vi "Hitrap_DiagnosticBoxGUI.panel.vi"() -> ()   [LabVIEW 2014, in "Hitrap_DiagnosticBoxGUI.lvlib"]
doc: "GUI for the DiagnosticBox class. It can be selected different step motors and perform a reference move to different diagnostics."
uses:
  Hitrap_DiagnosticBoxGUI.lvlib
  CSlibraries-extern/DimLVEvent/LVDimInterface/LVDimInterface.dim service type.ctl
  CSlibraries-extern/DimLVEvent/LVDimInterface/LVDimInterface.dic_info_service_notifier.vi
  CSCore/CSSystem/CoreLib/CoreLib.byte array 2 string.vi
  CSCore/CSSystem/CoreLib/CoreLib.int 2 byte array.vi
  CSCore/CSSystem/CoreLib/CoreLib.double 2 byte array.vi
  CSCore/CSSystem/CoreLib/CoreLib.lvlib
  CSlibraries/UtilityLib/UtilityLib.lvlib
  CSCore/GUIs/GOGUserGUIs/DeviceBaseGUI/DeviceBaseGUI.lvlib
  CSlibraries-extern/DimLVEvent/LVDimInterface/LVDimInterface.lvlib
  CSCore/BaseProcess/BaseProcess.lvlib
  CSCore/CSSystem/CSSystemLib/CSSystemLib.lvlib
panel:
  out "EMStop":bool
  out "loop 2":i32
  out "error out":errorcluster
  out "device state":bool
  out "error":bool=TRUE
  out "status":string
  out "pos error":bool
  out "status bit":u32(ring) items=["motorEnabled"=1, "negativeLimitSwitchActive"=2, "positiveLimitSwitchActive"=4, "limitSwitchesEnabled"=8, "limitSwitchesAreNormallyClosed"=16, "moving"=32, "referenced"=64, "inPosition"=128, "reserved2"=256, "reserved3"=512, "reserved4"=1024, "reserved5"=2048, "error"=4096, "reserved6"=8192, "reserved7"=16384, "reserved8"=32768, "user defined1"=65536, "user defined2"=131072, "user defined3"=262144, "user defined4"=524288, "user defined5"=1048576, "user defined6"=2097152, "user defined7"=4194304, "user defined8"=8388608, "user defined9"=16777216, "user defined10"=33554432, "user defined11"=67108864, "user defined12"=134217728, "user defined13"=268435456, "user defined14"=536870912, "user defined15"=1073741824, "user defined16"=2147483648]
  in  "Go Absolute":bool
  out "Moving":bool
  out "in Position":bool
  in  "steps to go":dbl
  out "loop 1":i32
  in  "error in (no error)":errorcluster
  in  "object ref":refnum<vi>
  in  "reset pos error":bool
  in  "Stop Movement":bool
  out "step count":dbl
  in  "Go Relative":bool
  out "Pos4Reached":bool
  in  "GoPosition4":bool
  in  "clear error":bool
  out "Enable":bool
  out "Pos3Reached":bool
  out "Pos2Reached":bool
  out "Pos1Reached":bool
  in  "GoPosition3":bool
  in  "GoPosition2":bool
  in  "GoPosition1":bool
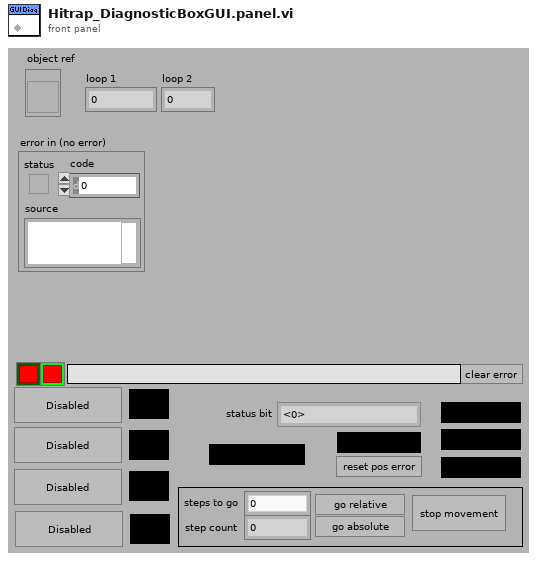
[diagram p1: front panel]
types:
  T1 = typedef "DeviceBaseGUI.lvlib/DeviceBaseGUI.i attribute.ctl" = cluster{"GOGFrontPanel.i attribute":T2}
  T2 = typedef "GOGFrontPanel.lvlib/GOGFrontPanel.i attribute.ctl" = cluster{"GOGObject":string, "Object":string, "Method":string, "Descriptor":T3, "Input Descriptor":string, "Output Descriptor":string, "inputNames":string[], "outputNames":string[], "Values":cluster{"descriptor":string, "value":string}[]}
  T3 = typedef "BaseProcess.lvlib/BaseProcess.descriptor string definition.ctl" = string
  T4 = cluster{"Diagnostic 1":string, "Diagnostic 2":string, "Diagnostic 3":string, "Diagnostic 4":string, "Diagnostic 5":string, "Position 1":dbl, "Position 2":dbl, "Position 3":dbl, "Position 4":dbl, "Position 5":dbl, "Reverse?":bool}
  T5 = enum8{"Enabled", "Disabled", "Disabled and Grayed Out"}
  T6 = typedef "LVDimInterface.lvlib/LVDimInterface.dim service type.ctl" = u16
  T7 = typedef "CoreDefs.call_type.ctl" = cluster{"Object":string, "Selector":string, "CallType":enum16{"simple", "synchronous", "asynchronous"}, "Async Object":string, "Async Selector":string, "Data Descriptor":T3, "Data":T8, "Error #":i32, "Expire":u32}
  T8 = typedef "CoreDefs.rawDataType.ctl" = i8[]
  T9 = typedef "MotorBase.lvlib/MotorBase.statusType.ctl" = u32
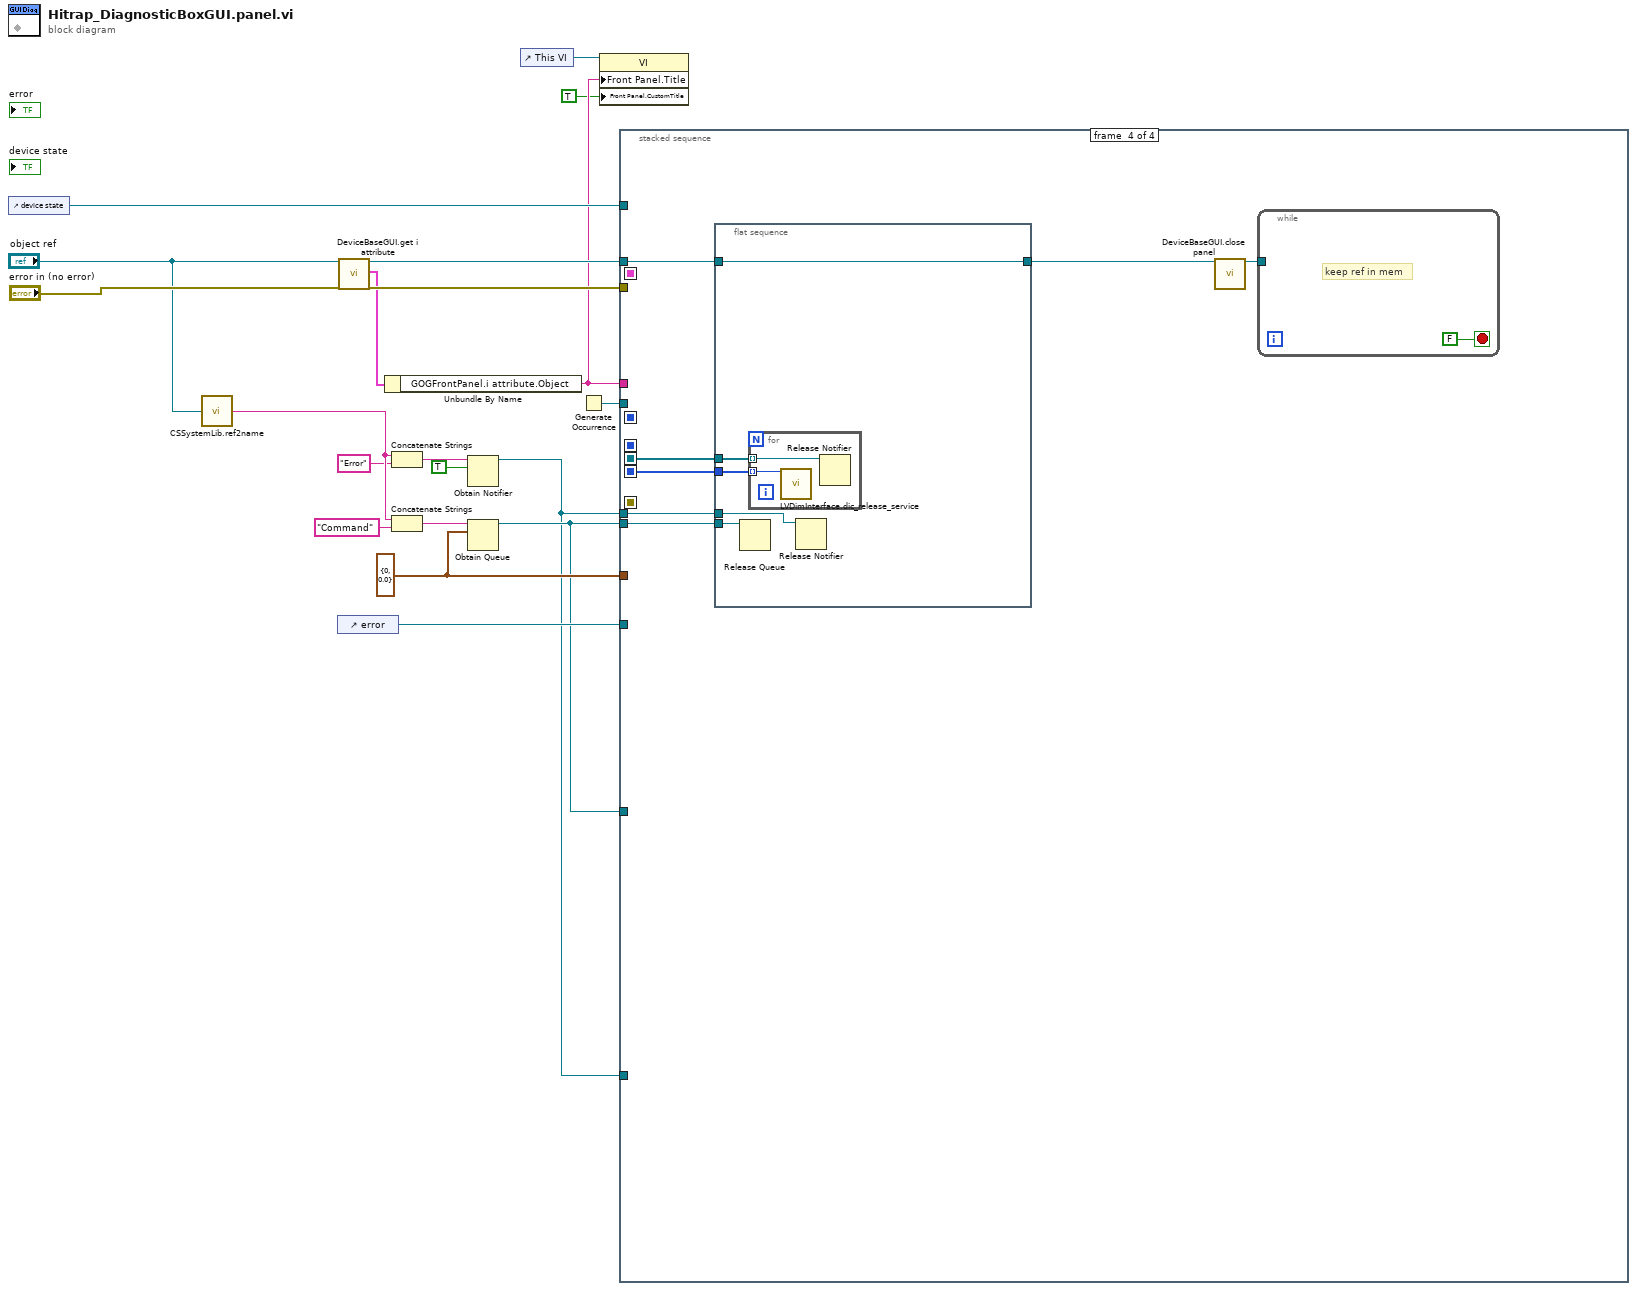
[diagram p0: block diagram]
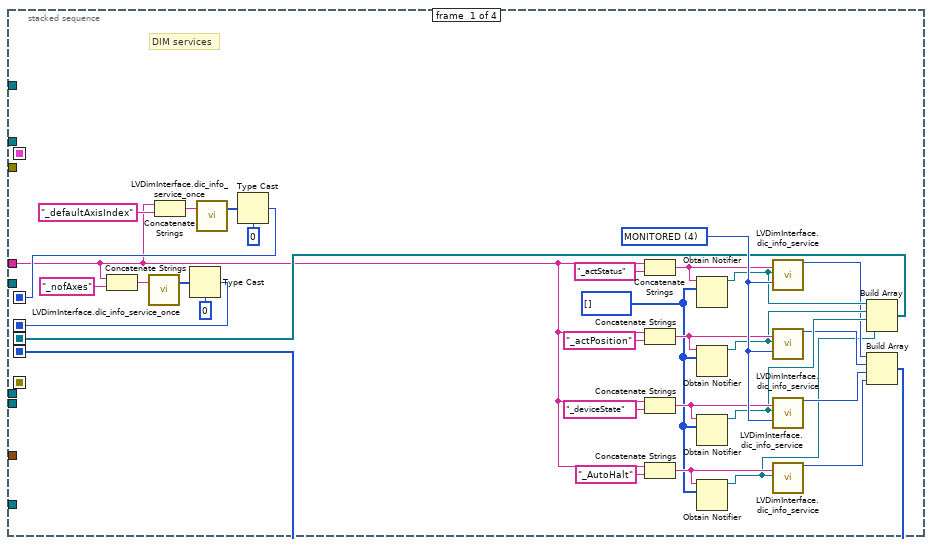
[diagram p2: hidden frame]
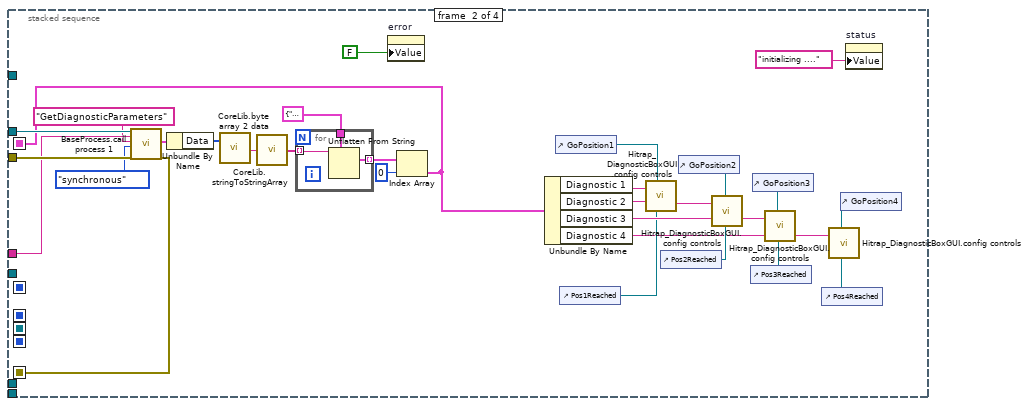
[diagram p3: hidden frame]
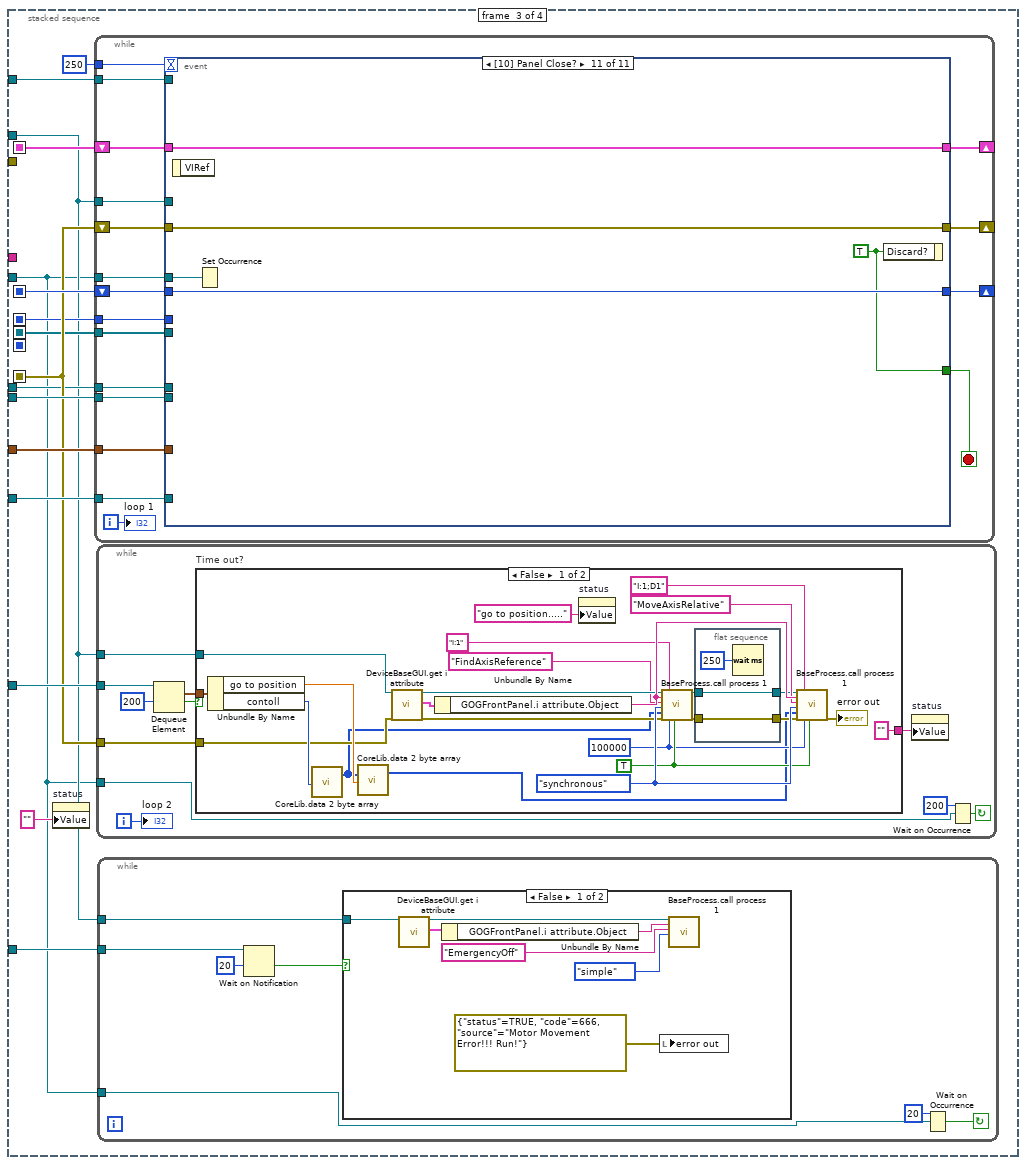
[diagram p4: hidden frame]
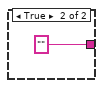
[diagram p6: hidden frame]
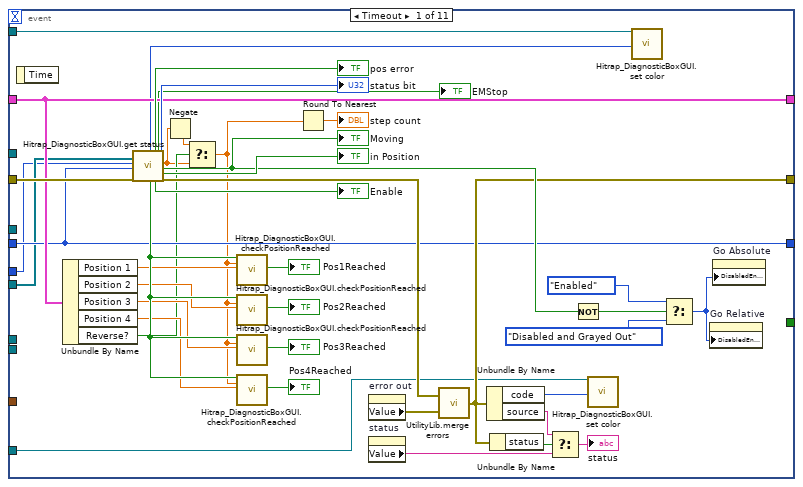
[diagram p7: hidden frame]
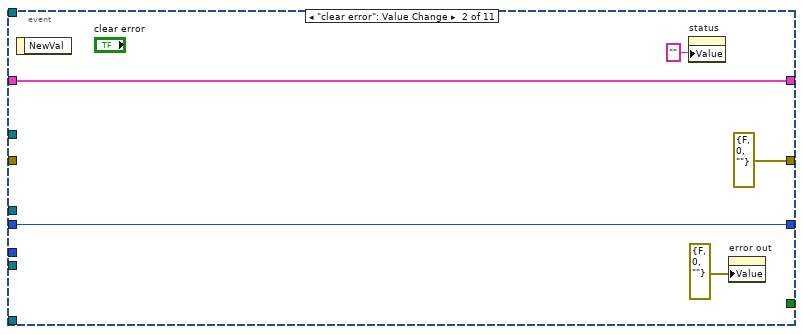
[diagram p8: hidden frame]
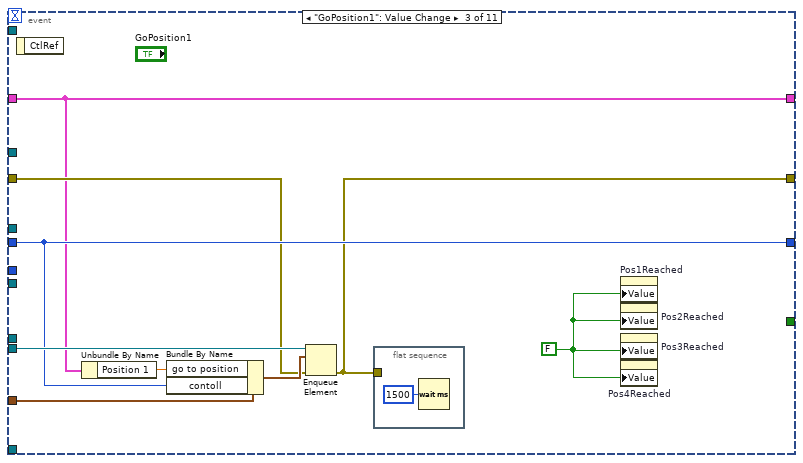
[diagram p9: hidden frame]
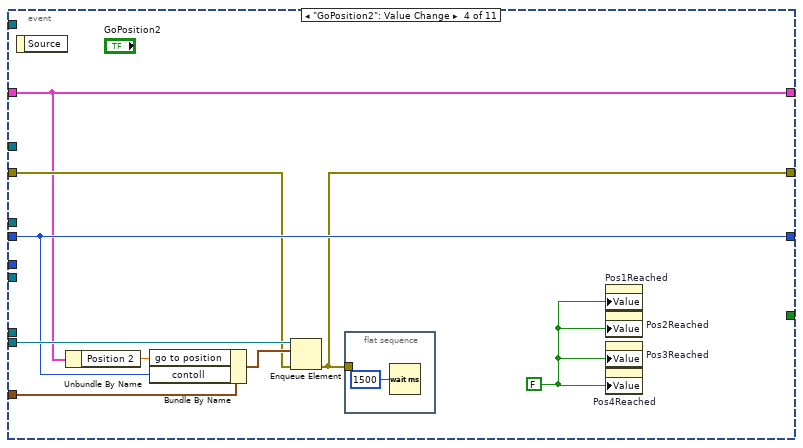
[diagram p10: hidden frame]
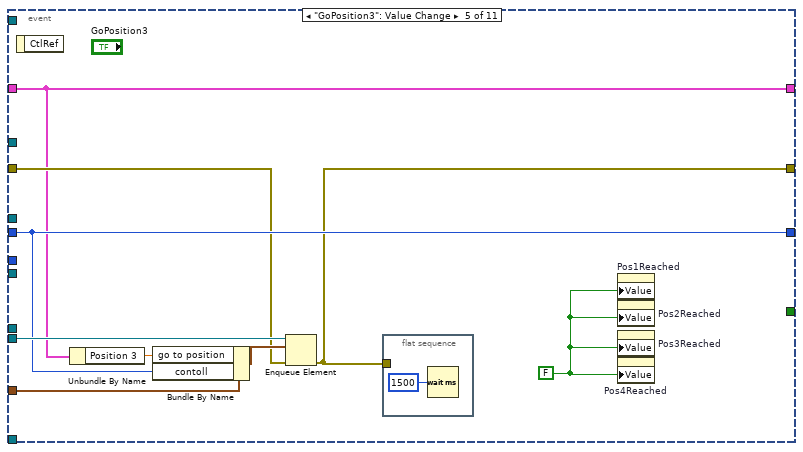
[diagram p11: hidden frame]
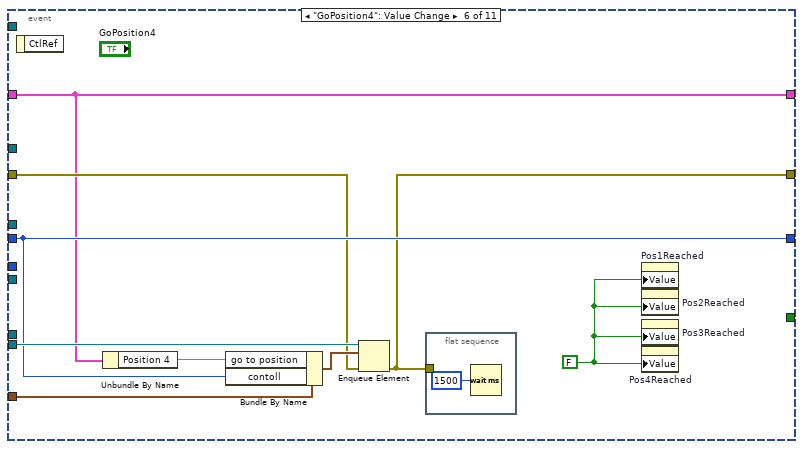
[diagram p12: hidden frame]
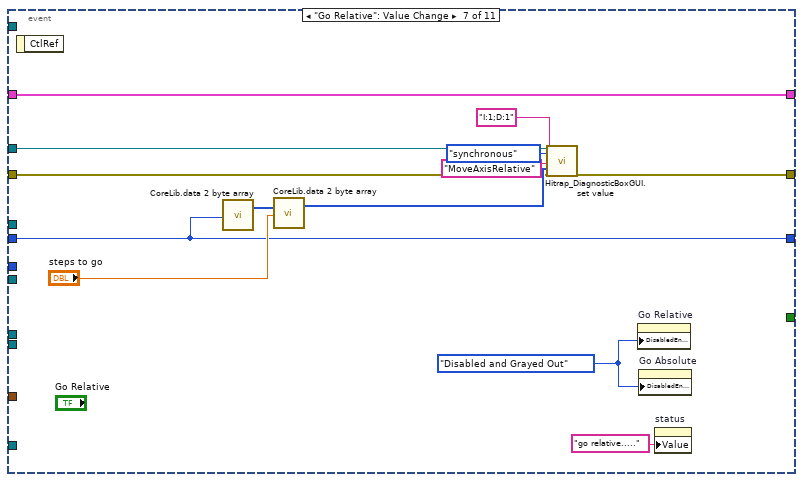
[diagram p13: hidden frame]
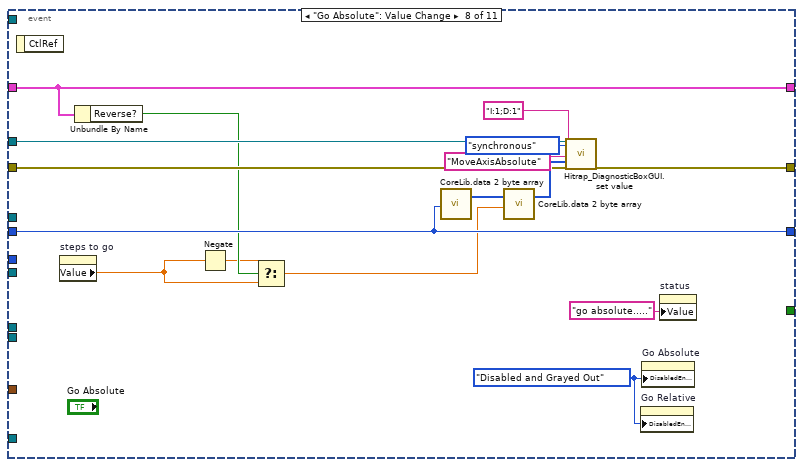
[diagram p14: hidden frame]
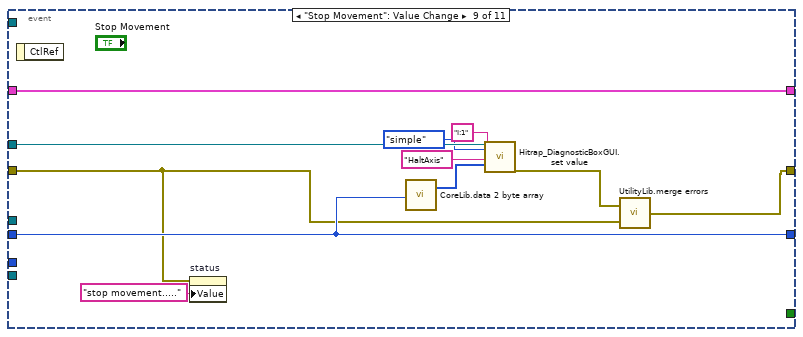
[diagram p15: hidden frame]
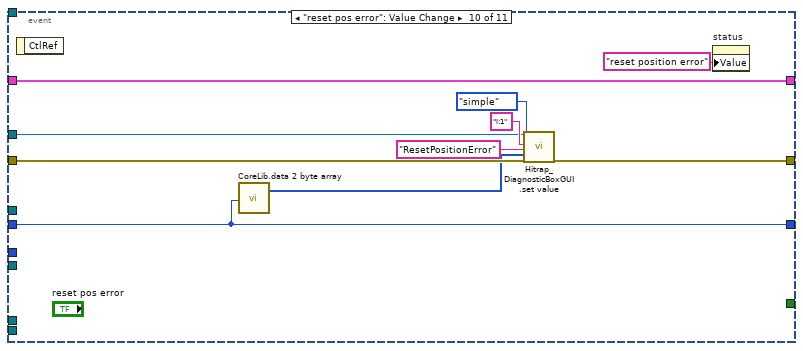
[diagram p16: hidden frame]
diagram:
  w18 = cluster{"contoll":i32, "go to position":dbl} {"contoll"=0, "go to position"=0.0} ("Cluster")
  n1 = control-ref of="device state"() -> (w20:refnum<vi>)
  n2 = call "CSSystemLib.ref2name.vi"("obj refnum"="object ref") -> ("name"=w5:string)
  n3 = control-ref of="error"() -> (w19:refnum<vi>)
  n4 = call "DeviceBaseGUI.get i attribute.vi"("i ref in"="object ref", "error in (no error)"="error in (no error)") -> ("i ref out"=w14:refnum<vi>, "i attribute"=w11:T1, "error out"=w12:errorcluster)  [unwired: 15 in]
  n5 = Unbundle By Name(w11) -> ("GOGFrontPanel.i attribute.Object"=w8:string)
  n6 = Concatenate Strings(w5, "Error" ("string")) -> (w6:string)
  n7 = Concatenate Strings(w5, "Command" ("name (unnamed)")) -> (w15:string)
  n8 = Obtain Notifier(name (unnamed)=w6, notification data type=TRUE) -> (notifier out=w2:refnum<notifier>)  [unwired: 2 in, 2 out]
  n9 = Obtain Queue(name (unnamed)=w15, element data type=w18) -> (queue out=w17:refnum<queue>)  [unwired: 3 in, 2 out]
  n10 = control-ref of="This VI"() -> (w9:refnum<vi>)
  n11 = Generate Occurrence() -> (w1:refnum<k4>)
  n12 = property class="VI"(reference=w9, "Front Panel.Title"=w8, "Front Panel.CustomTitle"=TRUE ("Front Panel Window:Custom Title")) -> ()  [unwired: 1 in, 2 out]
  n13 = stacked-sequence {
    seq-local: [w27 _ _ _] -> [_ _ w92 _]
    seq-local: [_ w52 _ _] -> [_ _ w90 _]
    seq-local: [_ w53 _ _] -> [_ _ w89 _]
    seq-local: [w40 _ _ _] -> [_ _ w88 _]
    seq-local: [w36 _ _ _] -> [_ _ w87 w316]
    seq-local: [w32 _ _ _] -> [_ _ _ w315]
    tunnel: w14 -> [_ w65 w84 w313]
    tunnel: w12 -> [_ w64 _ _]
    tunnel: w20 -> [_ _ w97 _]
    tunnel: w19 -> [_ _ w96 _]
    tunnel: w17 -> [_ _ w95 w317]
    tunnel: w18 -> [_ _ w94 _]
    tunnel: w17 -> [_ _ w93 _]
    tunnel: w8 -> [w24 w63 _ _]
    tunnel: w2 -> [_ _ w86 w312]
    tunnel: w2 -> [_ _ w85 _]
    tunnel: w1 -> [_ _ w83 _]
    frame #0 {
      w21 = i8[] []
      w51 = T6 4 items=["ONCE_ONLY"=1, "TIMED"=2, "MONITORED"=4] ("serviceType")
      # "DIM services"
      n14 = Concatenate Strings(w24, "_nofAxes" ("string")) -> (w47:string)
      n15 = call "LVDimInterface.dic_info_service_once.vi"("serviceName"=w47) -> ("data"=w45:i8[])  [unwired: 15 in, 3 out]
      n16 = Concatenate Strings(w24, "_defaultAxisIndex" ("string")) -> (w31:string)
      n17 = Type Cast(type=0, x=w45) -> (*(type *) &x=w40:i32)
      n18 = call "LVDimInterface.dic_info_service_once.vi"("serviceName"=w31) -> ("data"=w30:i8[])  [unwired: 15 in, 3 out]
      n19 = Type Cast(type=0, x=w30) -> (*(type *) &x=w27:i32)
      n20 = Concatenate Strings(w24, "_actStatus" ("string")) -> (w42:string)
      n21 = Concatenate Strings(w24, "_actPosition" ("string")) -> (w43:string)
      n22 = Concatenate Strings(w24, "_deviceState" ("string")) -> (w41:string)
      n23 = Concatenate Strings(w24, "_AutoHalt" ("string")) -> (w25:string)
      n24 = Obtain Notifier(name (unnamed)=w42, notification data type=w21) -> (notifier out=w39:refnum<notifier>)  [unwired: 2 in, 2 out]
      n25 = Obtain Notifier(name (unnamed)=w43, notification data type=w21) -> (notifier out=w38:refnum<notifier>)  [unwired: 2 in, 2 out]
      n26 = Obtain Notifier(name (unnamed)=w41, notification data type=w21) -> (notifier out=w37:refnum<notifier>)  [unwired: 2 in, 2 out]
      n27 = Obtain Notifier(name (unnamed)=w25, notification data type=w21) -> (notifier out=w22:refnum<notifier>)  [unwired: 2 in, 2 out]
      n28 = call-poly "LVDimInterface.dic_info_service.vi"("serviceName"=w42, "notifierRef"=w39, "serviceType"=w51) -> ("callBackID"=w35:i32)  [unwired: 15 in, 1 out]
      n29 = call-poly "LVDimInterface.dic_info_service.vi"("serviceName"=w43, "notifierRef"=w38, "serviceType"=w51) -> ("callBackID"=w34:i32)  [unwired: 15 in, 1 out]
      n30 = call-poly "LVDimInterface.dic_info_service.vi"("serviceName"=w41, "notifierRef"=w37, "serviceType"=w51) -> ("callBackID"=w33:i32)  [unwired: 15 in, 1 out]
      n31 = call-poly "LVDimInterface.dic_info_service.vi"("serviceName"=w25, "notifierRef"=w22) -> ("callBackID"=w23:i32)  [unwired: 16 in, 1 out]
      n32 = Build Array(w39, w38, w37, w22) -> (w36:refnum<notifier>[])
      n33 = Build Array(w35, w34, w33, w23) -> (w32:i32[])
    }
    frame #1 {
      n34 = call "BaseProcess.call process 1.vi"("i ref in"=w65, "Object"=w63, "Selector"="GetDiagnosticParameters", "CallType"=enum16{"simple", "synchronous", "asynchronous"}."synchronous", "error in (no error)"=w64) -> ("call cluster out"=w60:T7, "error out"=w52:errorcluster)  [unwired: 12 in, 1 out]
      n35 = Unbundle By Name(w60) -> ("Data"=w59:T8)
      n36 = call-poly "CoreLib.byte array 2 data.vi"("byteArray"=w59) -> ("string"=w58:string)  [unwired: 16 in, 2 out]
      n37 = call "CoreLib.stringToStringArray.vi"("String"=w58) -> ("Array"=w57:string[])
      n38 = for {
        tunnel: w57 -> [w82] mode=indexing
        tunnel: T4 {"Diagnostic 1"="", "Diagnostic 2"="", "Diagnostic 3"="", "Diagnostic 4"="", "Diagnostic 5"="", "Position 1"=0.0, "Position 2"=0.0, "Position 3"=0.0, "Position 4"=0.0, "Position 5"=0.0, "Reverse?"=FALSE} ("Diagnostic") -> [w81]
        tunnel: [w80] -> w55 mode=indexing
        n39 = Unflatten From String(type=w81, binary string=w82) -> (value=w80:T4)  [unwired: 3 in, 2 out]
      }
      n40 = property on="error" class="Bool (strict)"("Value"=FALSE ("status")) -> ()  [unwired: 2 in, 2 out]
      n41 = Index Array(array=w55, index=0) -> (element=w53:T4)
      n42 = Unbundle By Name(w53) -> ("Diagnostic 1"=w79:string, "Diagnostic 2"=w78:string, "Diagnostic 3"=w77:string, "Diagnostic 4"=w66:string)
      n43 = control-ref of="GoPosition1"() -> (w76:refnum<vi>)
      n44 = control-ref of="Pos1Reached"() -> (w75:refnum<vi>)
      n45 = call "Hitrap_DiagnosticBoxGUI.config controls.vi"("Text"=w79, "Refnum GO-Control"=w76, "Refnum Pos Reached Control"=w75) -> ()  [unwired: 17 in]
      n46 = control-ref of="Pos2Reached"() -> (w73:refnum<vi>)
      n47 = control-ref of="GoPosition2"() -> (w74:refnum<vi>)
      n48 = call "Hitrap_DiagnosticBoxGUI.config controls.vi"("Text"=w78, "Refnum GO-Control"=w74, "Refnum Pos Reached Control"=w73) -> ()  [unwired: 17 in]
      n49 = control-ref of="Pos3Reached"() -> (w71:refnum<vi>)
      n50 = control-ref of="GoPosition3"() -> (w72:refnum<vi>)
      n51 = call "Hitrap_DiagnosticBoxGUI.config controls.vi"("Text"=w77, "Refnum GO-Control"=w72, "Refnum Pos Reached Control"=w71) -> ()  [unwired: 17 in]
      n52 = control-ref of="Pos4Reached"() -> (w70:refnum<vi>)
      n53 = control-ref of="GoPosition4"() -> (w69:refnum<vi>)
      n54 = call "Hitrap_DiagnosticBoxGUI.config controls.vi"("Text"=w66, "Refnum GO-Control"=w69, "Refnum Pos Reached Control"=w70) -> ()  [unwired: 17 in]
      n55 = property on="status" class="Str"("Value"="initializing ...." ("source")) -> ()  [unwired: 2 in, 2 out]
    }
    frame #2 {
      n56 = property on="status" class="Str"("Value"="" ("status")) -> ()  [unwired: 2 in, 2 out]
      n57 = while {
        shift-right: [w168] -> _
        shift-left: w90 -> [w169]
        tunnel: 250 -> [w167]
        tunnel: w84 -> [w155]
        tunnel: w97 -> [w165]
        tunnel: w96 -> [w164]
        tunnel: w95 -> [w163]
        tunnel: w94 -> [w162]
        shift-right: [w161] -> _
        shift-left: w92 -> [w160]
        shift-right: [w158] -> _
        shift-left: w89 -> [w159]
        tunnel: w88 -> [w157]
        tunnel: w87 -> [w156]
        tunnel: w86 -> [w154]
        tunnel: w83 -> [w153]
        i -> [w166]
        stop <- w170 stop-if-true
        n58 = event shown="[10] Panel Close?" {
          selector: _ -> [_ _ _ _ _ _ _ _ _ _ _]
          dyn-events: _ -> [_ _ _ _ _ _ _ _ _ _ _]
          timeout: w167 -> [_ _ _ _ _ _ _ _ _ _ _]
          tunnel: [_ _ _ _ _ _ _ _ _ _ w306] -> w170
          tunnel: w169 -> [w199 _ w219 w229 w239 w249 w260 w278 w285 w302 w310]
          tunnel: [w190 errorcluster {"status"=FALSE, "code"=0, "source"=""} ("error out") w218 w228 w238 w248 w268 w284 w293 w301 w310] -> w168
          tunnel: w155 -> [_ _ _ _ _ _ w259 w277 w295 w303 _]
          tunnel: w165 -> [w181 _ _ _ _ _ _ _ _ _ _]
          tunnel: w164 -> [w180 _ _ _ _ _ _ _ _ _ _]
          tunnel: w163 -> [_ _ w223 w232 w242 w253 _ _ _ _ _]
          tunnel: w162 -> [_ _ w222 w231 w241 w252 _ _ _ _ _]
          tunnel: w160 -> [w183 w213 w220 w230 w240 w250 w261 w280 w292 w298 w309]
          tunnel: [w183 w213 w220 w230 w240 w250 w261 w280 w292 w298 w309] -> w161
          tunnel: w159 -> [w184 w211 w216 w226 w236 w246 w265 w273 w291 w299 w308]
          tunnel: [w184 w211 w216 w226 w236 w246 w265 w273 w291 w299 w308] -> w158
          tunnel: w157 -> [w177 _ _ _ _ _ _ _ _ _ _]
          tunnel: w156 -> [w178 _ _ _ _ _ _ _ _ _ _]
          tunnel: w154 -> [_ _ _ _ _ _ _ _ _ _ _]
          tunnel: w153 -> [_ _ _ _ _ _ _ _ _ _ w307]
          event Timeout {
            n59 = event-data() -> ()  [unwired: 1 in, 1 out]
            n60 = Unbundle By Name(w184) -> ("Position 1"=w188:dbl, "Position 2"=w187:dbl, "Position 3"=w186:dbl, "Position 4"=w185:dbl, "Reverse?"=w176:bool)
            n61 = call "Hitrap_DiagnosticBoxGUI.get status.vi"("DIMArray"=w178, "NofAxes"=w177, "Axis"=w183, "error in (no error)"=w199) -> ("deviceState"=w182:i32, "Reference"=w189:bool, "Error"=→"pos error":bool, "Enable"=→"Enable":bool, "AutoHalt?"=→"EMStop":bool, "actValueStatu"=→"status bit":T9, "Position"=w175:dbl, "Moving"=w200:bool, "in Position"=→"in Position":bool, "error out"=w191:errorcluster)  [unwired: 6 in]
            "Moving" <- w200
            n62 = Negate(x=w175) -> (-x=w174:dbl)
            n63 = Select(t=w174, s=w176, f=w175) -> (s? t:f=w173:dbl)
            n64 = call "Hitrap_DiagnosticBoxGUI.checkPositionReached.vi"("referenced?"=w189, "actPosition []"=w173, "desired Position"=w188) -> ("Position Reached?"=→"Pos1Reached":bool)  [unwired: 16 in]
            n65 = call "Hitrap_DiagnosticBoxGUI.checkPositionReached.vi"("referenced?"=w189, "actPosition []"=w173, "desired Position"=w187) -> ("Position Reached?"=→"Pos2Reached":bool)  [unwired: 16 in]
            n66 = call "Hitrap_DiagnosticBoxGUI.checkPositionReached.vi"("referenced?"=w189, "actPosition []"=w173, "desired Position"=w186) -> ("Position Reached?"=→"Pos3Reached":bool)  [unwired: 16 in]
            n67 = call "Hitrap_DiagnosticBoxGUI.checkPositionReached.vi"("referenced?"=w189, "actPosition []"=w173, "desired Position"=w185) -> ("Position Reached?"=→"Pos4Reached":bool)  [unwired: 16 in]
            n68 = Round To Nearest(number=w173) -> (nearest integer value=→"step count":dbl)
            n69 = property on="error out" class="Clust (strict)"() -> ("Value"=w196:errorcluster)  [unwired: 2 in, 2 out]
            n70 = property on="status" class="Str"() -> ("Value"=w193:string)  [unwired: 2 in, 2 out]
            n71 = call "UtilityLib.merge errors.vi"("error2 (no error)"=w196, "error1 (no error)"=w191) -> ("error out"=w190:errorcluster)
            n72 = Unbundle By Name(w190) -> ("code"=w179:i32, "source"=w194:string)
            n73 = Unbundle By Name(w190) -> ("status"=w195:bool)
            n74 = Select(t=w194, s=w195, f=w193) -> (s? t:f=→"status":string)
            n75 = Not(x=w200) -> (.not. x?=w201:bool)
            n76 = call "Hitrap_DiagnosticBoxGUI.set color.vi"("button"=w180, "Numeric"=w179) -> ()  [unwired: 17 in, 1 out]
            n77 = call "Hitrap_DiagnosticBoxGUI.set color.vi"("button"=w181, "Numeric"=w182) -> ()  [unwired: 17 in, 1 out]
            n78 = Select(t=T5."Enabled" ("Disabled"), s=w201, f=T5."Disabled and Grayed Out" ("Disabled")) -> (s? t:f=w202:T5)
            n79 = property on="Go Relative" class="Bool"("DisabledEnum"=w202) -> ()  [unwired: 2 in, 2 out]
            n80 = property on="Go Absolute" class="Bool"("DisabledEnum"=w202) -> ()  [unwired: 2 in, 2 out]
          }
          event "clear error": Value Change {
            n81 = event-data() -> ()  [unwired: 1 in, 1 out]
            n82 = property on="status" class="Str"("Value"="" ("status")) -> ()  [unwired: 2 in, 2 out]
            n83 = property on="error out" class="Clust (strict)"("Value"=errorcluster {"status"=FALSE, "code"=0, "source"=""} ("error out")) -> ()  [unwired: 2 in, 2 out]
          }
          event "GoPosition1": Value Change {
            w224 = FALSE ("OutReached")
            n84 = event-data() -> ()  [unwired: 1 in, 1 out]
            n85 = Unbundle By Name(w216) -> ("Position 1"=w217:dbl)
            n86 = Bundle By Name(cluster=w222, "go to position"=w217, "contoll"=w220) -> (w221:cluster{"contoll":i32, "go to position":dbl})
            n87 = Enqueue Element(queue=w223, element=w221, error in (no error)=w219) -> (error out=w218:errorcluster)  [unwired: 1 in, 2 out]
            n88 = flat-sequence {
              tunnel: w218 -> [_]
              frame #0 {
                n89 = Wait (ms)(milliseconds to wait=u32 1500) -> ()  [unwired: 1 out]
              }
            }
            n90 = property on="Pos1Reached" class="Bool (strict)"("Value"=w224) -> ()  [unwired: 2 in, 2 out]
            n91 = property on="Pos2Reached" class="Bool (strict)"("Value"=w224) -> ()  [unwired: 2 in, 2 out]
            n92 = property on="Pos3Reached" class="Bool (strict)"("Value"=w224) -> ()  [unwired: 2 in, 2 out]
            n93 = property on="Pos4Reached" class="Bool (strict)"("Value"=w224) -> ()  [unwired: 2 in, 2 out]
          }
          event "GoPosition2": Value Change {
            w234 = FALSE ("OutReached")
            n94 = event-data() -> ()  [unwired: 1 in, 1 out]
            n95 = Unbundle By Name(w226) -> ("Position 2"=w227:dbl)
            n96 = Bundle By Name(cluster=w231, "go to position"=w227, "contoll"=w230) -> (w233:cluster{"contoll":i32, "go to position":dbl})
            n97 = Enqueue Element(queue=w232, element=w233, error in (no error)=w229) -> (error out=w228:errorcluster)  [unwired: 1 in, 2 out]
            n98 = flat-sequence {
              tunnel: w228 -> [_]
              frame #0 {
                n99 = Wait (ms)(milliseconds to wait=u32 1500) -> ()  [unwired: 1 out]
              }
            }
            n100 = property on="Pos1Reached" class="Bool (strict)"("Value"=w234) -> ()  [unwired: 2 in, 2 out]
            n101 = property on="Pos2Reached" class="Bool (strict)"("Value"=w234) -> ()  [unwired: 2 in, 2 out]
            n102 = property on="Pos3Reached" class="Bool (strict)"("Value"=w234) -> ()  [unwired: 2 in, 2 out]
            n103 = property on="Pos4Reached" class="Bool (strict)"("Value"=w234) -> ()  [unwired: 2 in, 2 out]
          }
          event "GoPosition3": Value Change {
            w244 = FALSE ("OutReached")
            n104 = event-data() -> ()  [unwired: 1 in, 1 out]
            n105 = Unbundle By Name(w236) -> ("Position 3"=w237:dbl)
            n106 = Bundle By Name(cluster=w241, "go to position"=w237, "contoll"=w240) -> (w243:cluster{"contoll":i32, "go to position":dbl})
            n107 = Enqueue Element(queue=w242, element=w243, error in (no error)=w239) -> (error out=w238:errorcluster)  [unwired: 1 in, 2 out]
            n108 = flat-sequence {
              tunnel: w238 -> [_]
              frame #0 {
                n109 = Wait (ms)(milliseconds to wait=u32 1500) -> ()  [unwired: 1 out]
              }
            }
            n110 = property on="Pos1Reached" class="Bool (strict)"("Value"=w244) -> ()  [unwired: 2 in, 2 out]
            n111 = property on="Pos2Reached" class="Bool (strict)"("Value"=w244) -> ()  [unwired: 2 in, 2 out]
            n112 = property on="Pos3Reached" class="Bool (strict)"("Value"=w244) -> ()  [unwired: 2 in, 2 out]
            n113 = property on="Pos4Reached" class="Bool (strict)"("Value"=w244) -> ()  [unwired: 2 in, 2 out]
          }
          event "GoPosition4": Value Change {
            w254 = FALSE ("OutReached")
            n114 = event-data() -> ()  [unwired: 1 in, 1 out]
            n115 = Unbundle By Name(w246) -> ("Position 4"=w247:dbl)
            n116 = Bundle By Name(cluster=w252, "go to position"=w247, "contoll"=w250) -> (w251:cluster{"contoll":i32, "go to position":dbl})
            n117 = Enqueue Element(queue=w253, element=w251, error in (no error)=w249) -> (error out=w248:errorcluster)  [unwired: 1 in, 2 out]
            n118 = flat-sequence {
              tunnel: w248 -> [_]
              frame #0 {
                n119 = Wait (ms)(milliseconds to wait=u32 1500) -> ()  [unwired: 1 out]
              }
            }
            n120 = property on="Pos1Reached" class="Bool (strict)"("Value"=w254) -> ()  [unwired: 2 in, 2 out]
            n121 = property on="Pos2Reached" class="Bool (strict)"("Value"=w254) -> ()  [unwired: 2 in, 2 out]
            n122 = property on="Pos3Reached" class="Bool (strict)"("Value"=w254) -> ()  [unwired: 2 in, 2 out]
            n123 = property on="Pos4Reached" class="Bool (strict)"("Value"=w254) -> ()  [unwired: 2 in, 2 out]
          }
          event "Go Relative": Value Change {
            w267 = T5."Disabled and Grayed Out" ("Disabled")
            n124 = event-data() -> ()  [unwired: 1 in, 1 out]
            n125 = call-poly "CoreLib.data 2 byte array.vi"("i32"=w261) -> ("byteArray out"=w264:T8)  [unwired: 18 in]
            n126 = call-poly "CoreLib.data 2 byte array.vi"("byteArray"=w264, "f64"="steps to go") -> ("byteArray out"=w262:T8)  [unwired: 17 in]
            n127 = call "Hitrap_DiagnosticBoxGUI.set value.vi"("i ref in"=w259, "CallType"=enum16{"simple", "synchronous", "asynchronous"}."synchronous", "Data Discriptor"="I:1;D:1", "Selector"="MoveAxisRelative", "Data"=w262, "error in (no error)"=w260) -> ("error out"=w268:errorcluster)  [unwired: 13 in]
            n128 = property on="Go Relative" class="Bool"("DisabledEnum"=w267) -> ()  [unwired: 2 in, 2 out]
            n129 = property on="Go Absolute" class="Bool"("DisabledEnum"=w267) -> ()  [unwired: 2 in, 2 out]
            n130 = property on="status" class="Str"("Value"="go relative....." ("status")) -> ()  [unwired: 2 in, 2 out]
          }
          event "Go Absolute": Value Change {
            w283 = T5."Disabled and Grayed Out" ("Disabled")
            n131 = event-data() -> ()  [unwired: 1 in, 1 out]
            n132 = property on="steps to go" class="DigNum (strict)"() -> ("Value"=w269:dbl)  [unwired: 2 in, 2 out]
            n133 = Unbundle By Name(w273) -> ("Reverse?"=w272:bool)
            n134 = Negate(x=w269) -> (-x=w270:dbl)
            n135 = Select(t=w270, s=w272, f=w269) -> (s? t:f=w271:dbl)
            n136 = call-poly "CoreLib.data 2 byte array.vi"("i32"=w280) -> ("byteArray out"=w279:T8)  [unwired: 18 in]
            n137 = call-poly "CoreLib.data 2 byte array.vi"("byteArray"=w279, "f64"=w271) -> ("byteArray out"=w281:T8)  [unwired: 17 in]
            n138 = call "Hitrap_DiagnosticBoxGUI.set value.vi"("i ref in"=w277, "CallType"=enum16{"simple", "synchronous", "asynchronous"}."synchronous", "Data Discriptor"="I:1;D:1", "Selector"="MoveAxisAbsolute", "Data"=w281, "error in (no error)"=w278) -> ("error out"=w284:errorcluster)  [unwired: 13 in]
            n139 = property on="Go Relative" class="Bool"("DisabledEnum"=w283) -> ()  [unwired: 2 in, 2 out]
            n140 = property on="Go Absolute" class="Bool"("DisabledEnum"=w283) -> ()  [unwired: 2 in, 2 out]
            n141 = property on="status" class="Str"("Value"="go absolute....." ("status")) -> ()  [unwired: 2 in, 2 out]
          }
          event "Stop Movement": Value Change {
            n142 = event-data() -> ()  [unwired: 1 in, 1 out]
            n143 = property on="status" class="Str"(error in=w285, "Value"="stop movement....." ("status")) -> ()  [unwired: 1 in, 2 out]
            n144 = call-poly "CoreLib.data 2 byte array.vi"("i32"=w292) -> ("byteArray out"=w287:T8)  [unwired: 18 in]
            n145 = call "Hitrap_DiagnosticBoxGUI.set value.vi"("i ref in"=w295, "CallType"=enum16{"simple", "synchronous", "asynchronous"}."simple", "Data Discriptor"="I:1", "Selector"="HaltAxis", "Data"=w287) -> ("error out"=w288:errorcluster)  [unwired: 14 in]
            n146 = call "UtilityLib.merge errors.vi"("error2 (no error)"=w285, "error1 (no error)"=w288) -> ("error out"=w293:errorcluster)
          }
          event "reset pos error": Value Change {
            n147 = event-data() -> ()  [unwired: 1 in, 1 out]
            n148 = call-poly "CoreLib.data 2 byte array.vi"("i32"=w298) -> ("byteArray out"=w297:T8)  [unwired: 18 in]
            n149 = call "Hitrap_DiagnosticBoxGUI.set value.vi"("i ref in"=w303, "CallType"=enum16{"simple", "synchronous", "asynchronous"}."simple", "Data Discriptor"="I:1", "Selector"="ResetPositionError", "Data"=w297, "error in (no error)"=w302) -> ("error out"=w301:errorcluster)  [unwired: 13 in]
            n150 = property on="status" class="Str"("Value"="reset position error" ("status")) -> ()  [unwired: 2 in, 2 out]
          }
          event Panel Close? {
            w306 = TRUE ("Discard?")
            n151 = event-data() -> ()  [unwired: 1 in, 1 out]
            n152 = Set Occurrence(w307) -> ()
            n153 = event-data("Discard?"=w306) -> ()  [unwired: 1 in, 1 out]
          }
        }
        "loop 1" <- w166
      }
      n154 = while {
        tunnel: w93 -> [w122]
        tunnel: w84 -> [w121]
        tunnel: w90 -> [w119]
        tunnel: w83 -> [w113]
        i -> [w117]
        stop <- w114 continue-if-true
        n155 = Dequeue Element(queue=w122, timeout in ms (-1)=200) -> (element=w123:cluster{"contoll":i32, "go to position":dbl}, timed out?=w120:bool)  [unwired: 1 in, 2 out]
        n156 = case "Time out?" shown="False" w120 {
          tunnel: w123 -> [w148 _]
          tunnel: w121 -> [w135 _]
          tunnel: w119 -> [w134 _]
          tunnel: ["" ("status") "" ("status")] -> w116
          frame False {
            w142 = enum16{"simple", "synchronous", "asynchronous"}."synchronous" ("CallType")
            w139 = 100000 ("timeout (ms)")
            w140 = TRUE ("expire")
            n157 = Unbundle By Name(w148) -> ("go to position"=w145:dbl, "contoll"=w146:i32)
            n158 = call-poly "CoreLib.data 2 byte array.vi"("i32"=w146) -> ("byteArray out"=w125:T8)  [unwired: 18 in]
            n159 = call-poly "CoreLib.data 2 byte array.vi"("byteArray"=w125, "f64"=w145) -> ("byteArray out"=w124:T8)  [unwired: 17 in]
            n160 = call "DeviceBaseGUI.get i attribute.vi"("i ref in"=w135, "error in (no error)"=w134) -> ("i ref out"=w136:refnum<vi>, "i attribute"=w138:T1, "error out"=w137:errorcluster)  [unwired: 15 in]
            n161 = Unbundle By Name(w138) -> ("GOGFrontPanel.i attribute.Object"=w141:string)
            n162 = property on="status" class="Str"("Value"="go to position....." ("status")) -> ()  [unwired: 2 in, 2 out]
            n163 = call "BaseProcess.call process 1.vi"("i ref in"=w136, "Object"=w141, "Selector"="FindAxisReference" ("Data Discriptor"), "CallType"=w142, "Data"=w125, "error in (no error)"=w137, "Data Descriptor"="I:1" ("Data Discriptor"), "timeout (ms)"=w139, "expire"=w140) -> ("i ref out"=w130:refnum<vi>, "error out"=w129:errorcluster)  [unwired: 8 in, 1 out]
            n164 = flat-sequence {
              tunnel: w130 -> [w151]
              tunnel: w129 -> [w150]
              tunnel: [w151] -> w128
              tunnel: [w150] -> w127
              frame #0 {
                n165 = Wait (ms)(milliseconds to wait=u32 250) -> ()  [unwired: 1 out]
              }
            }
            n166 = call "BaseProcess.call process 1.vi"("i ref in"=w128, "Object"=w141, "Selector"="MoveAxisRelative" ("Data Discriptor"), "CallType"=w142, "Data"=w124, "error in (no error)"=w127, "Data Descriptor"="I:1;D1" ("Data Discriptor"), "timeout (ms)"=w139, "expire"=w140) -> ("error out"=→"error out":errorcluster)  [unwired: 8 in, 2 out]
          }
          frame True {
          }
        }
        n167 = property on="status" class="Str"("Value"=w116) -> ()  [unwired: 2 in, 2 out]
        n168 = Wait on Occurrence(2:w113, 3:200 ("ms timeout (-1)")) -> (0:w114:bool)  [unwired: 1 in]
        "loop 2" <- w117
      }
      n169 = while {
        tunnel: w85 -> [w105]
        tunnel: w84 -> [w102]
        tunnel: w83 -> [w100]
        stop <- w101 continue-if-true
        n170 = Wait on Notification(notifier=w105, timeout in ms (-1)=20) -> (timed out?=w103:bool)  [unwired: 2 in, 3 out]
        n171 = case shown="False" w103 {
          tunnel: w102 -> [w109 _]
          frame False {
            n172 = call "DeviceBaseGUI.get i attribute.vi"("i ref in"=w109) -> ("i ref out"=w111:refnum<vi>, "i attribute"=w112:T1)  [unwired: 16 in, 1 out]
            n173 = Unbundle By Name(w112) -> ("GOGFrontPanel.i attribute.Object"=w110:string)
            n174 = local write "error out"(errorcluster {"status"=TRUE, "code"=666, "source"="Motor Movement Error!!! Run!"} ("error out")) -> ()
            n175 = call "BaseProcess.call process 1.vi"("i ref in"=w111, "Object"=w110, "Selector"="EmergencyOff", "CallType"=enum16{"simple", "synchronous", "asynchronous"}."simple") -> ()  [unwired: 13 in, 3 out]
          }
          frame True {
          }
        }
        n176 = Wait on Occurrence(2:w100, 3:20 ("ms timeout (-1)")) -> (0:w101:bool)  [unwired: 1 in]
      }
    }
    frame #3 {
      n177 = flat-sequence {
        tunnel: w317 -> [w320]
        tunnel: w316 -> [w323]
        tunnel: w315 -> [w322]
        tunnel: [w321] -> w314
        tunnel: w313 -> [w321]
        tunnel: w312 -> [w319]
        frame #0 {
          n178 = Release Queue(queue=w320) -> ()  [unwired: 2 in, 3 out]
          n179 = for {
            tunnel: w323 -> [w325] mode=indexing
            tunnel: w322 -> [w324] mode=indexing
            n180 = call "LVDimInterface.dic_release_service.vi"("callBackID"=w324) -> ()  [unwired: 18 in, 1 out]
            n181 = Release Notifier(notifier=w325) -> ()  [unwired: 2 in, 3 out]
          }
          n182 = Release Notifier(notifier=w319) -> ()  [unwired: 2 in, 3 out]
        }
      }
      n183 = call "DeviceBaseGUI.close panel.vi"("i ref in"=w314) -> ("i ref out"=w311:refnum<vi>)  [unwired: 17 in, 1 out]
      n184 = while {
        tunnel: w311 -> [_]
        stop <- FALSE stop-if-true
        # "keep ref in mem"
      }
    }
  }
